vi "asyncAcq_occurenceRef.vi"(0 "reference":refnum<class "OSA.lvclass">, 2 "spectrIdx in":u16, 3 "acqType in":u32, 4 "error in":u32, 5 "error in (no error)":errorcluster, 7 "action":T1) -> (14 "duplicate reference":refnum<class "OSA.lvclass">, 19 "error out":errorcluster)   [LabVIEW 2010, in "OSA.lvclass"]
doc: "Reads the contents of a <B>Thorlabs_OSA_64</B> object.\n\n[GOOP 1.0]"
uses:
  OSA.lvclass
  asyncAcq_occRef_action.ctl
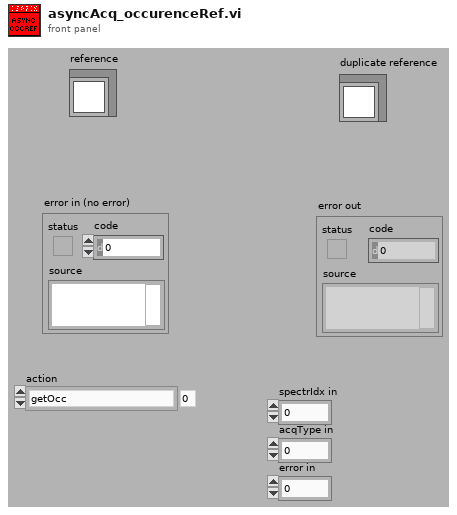
[diagram p1: front panel]
types:
  T1 = typedef "OSA.lvclass/asyncAcq_occRef_action.ctl" = enum16{"getOcc", "getAcqPars", "setOcc", "setAcqPars"}
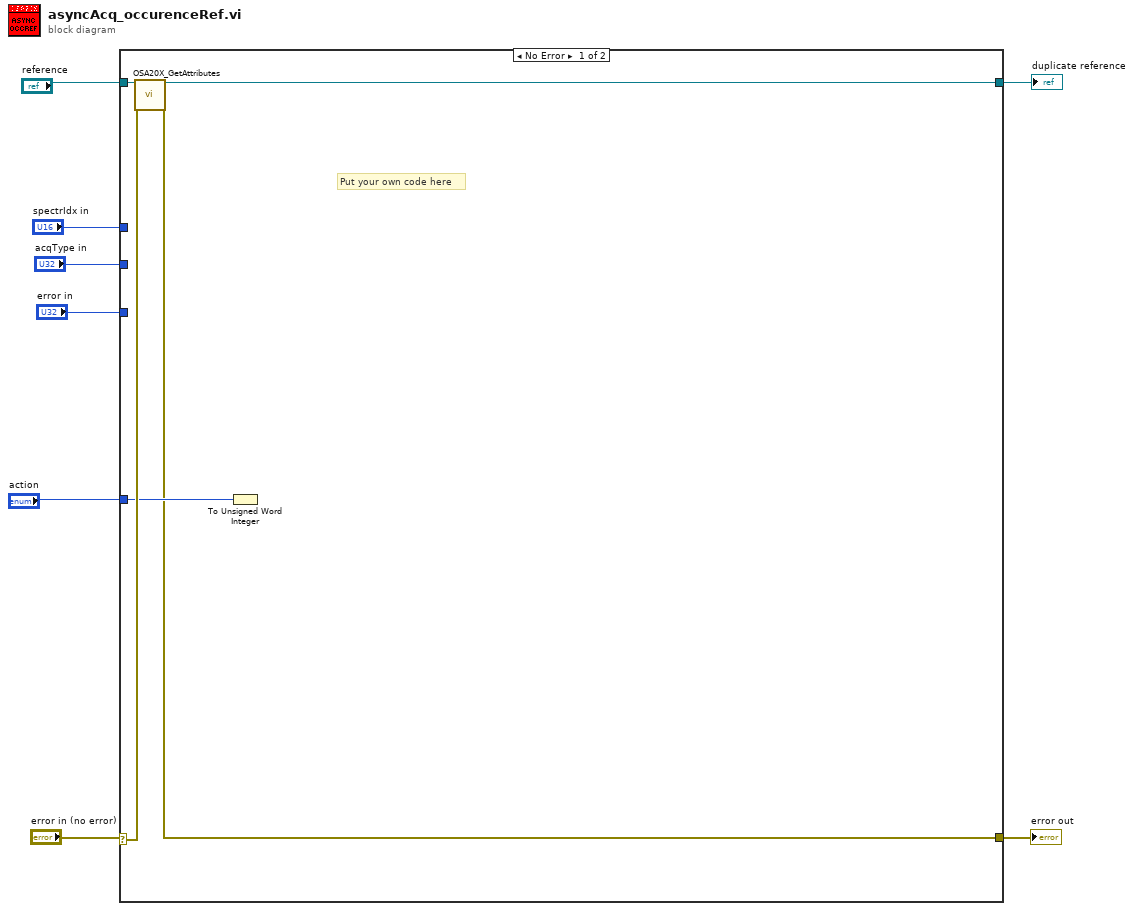
[diagram p0: block diagram]
diagram:
  n1 = case shown="No Error" "error in (no error)" {
    selector: "error in (no error)" -> [w11 w14]
    tunnel: [w9 w14] -> w8
    tunnel: "reference" -> [w13 w15]
    tunnel: [w12 w15] -> w5
    tunnel: "action" -> [w10 _]
    tunnel: "spectrIdx in" -> [_ _]
    tunnel: "acqType in" -> [_ _]
    tunnel: "error in" -> [_ _]
    frame No Error {
      # "Put your own code here"
      n2 = call "OSA20X_GetAttributes.vi"("reference in"=w13, "error in (no error)"=w11) -> ("reference out"=w12:refnum<class "OSA.lvclass">, "error out"=w9:errorcluster)  [unwired: 14 in, 2 out]
      n3 = To Unsigned Word Integer(number=w10) -> ()  [unwired: 1 out]
    }
    frame Error {
      # "Error"
    }
  }
  "error out" <- w8
  "duplicate reference" <- w5
